vi "Send Message.vi"(8 "error in (no error)":errorcluster, 10 "Message.lvclass":refnum<class "Message.lvclass">, 11 "Message Transport in":refnum<class "Message Transport.lvclass">) -> (0 "error out":errorcluster, 3 "Message Transport out":refnum<class "Message Transport.lvclass">)   [LabVIEW 2018, in "Message Transport.lvclass"]
uses:
  Message Transport.lvclass
  Message_class/Message.lvclass
  Message Transport.lvclass/Message Transport.ctl
  Communication_class/Get Message Queue.vi
  Communication_class/Set Message Queue.vi
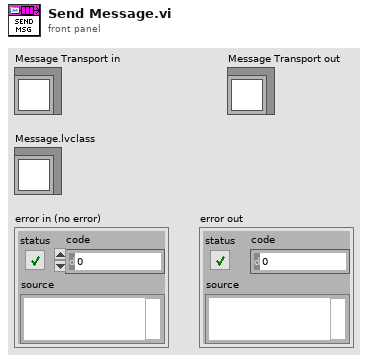
[diagram p1: front panel]
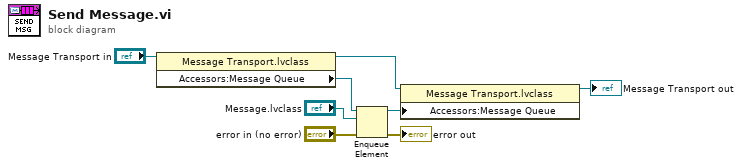
[diagram p0: block diagram]
diagram:
  n1 = property class="Message Transport.lvclass"(reference="Message Transport in") -> (reference out=w5:refnum<class "Message Transport.lvclass">, "Accessors:Message Queue"=w3:refnum<queue>)  [unwired: 1 in, 1 out]
  n2 = Enqueue Element(queue=w3, element="Message.lvclass", error in (no error)="error in (no error)") -> (queue out=w2:refnum<queue>, error out=→"error out":errorcluster)  [unwired: 1 in, 1 out]
  n3 = property class="Message Transport.lvclass"(reference=w5, "Accessors:Message Queue"=w2) -> (reference out=→"Message Transport out":refnum<class "Message Transport.lvclass">)  [unwired: 1 in, 1 out]
